vi "convertPhysicalChannels.vi"(8 "error in (no error)":errorcluster, 10 "physicalChannels":string[](array[string]), 11 "K2602 in":refnum<class "K2602.lvclass">) -> (0 "error out":errorcluster, 2 "channel":i32[](array[numeric]), 3 "K2602 out":refnum<class "K2602.lvclass">)   [LabVIEW 2011, in "Hardware.lvlib" / "Channels.lvlib" / "K2602.lvclass"]
uses:
  K2602.lvclass
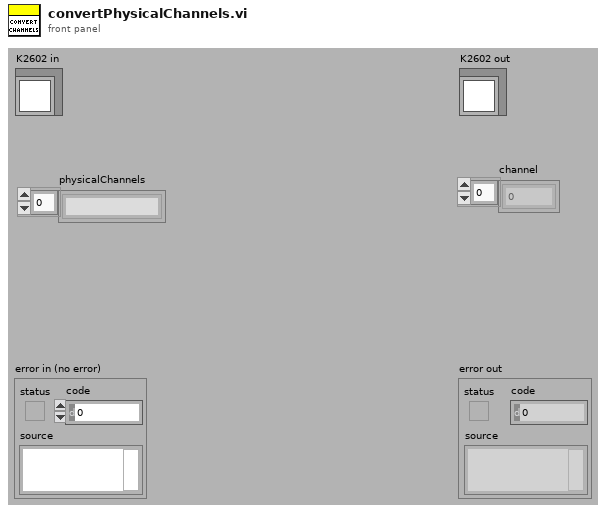
[diagram p1: front panel]
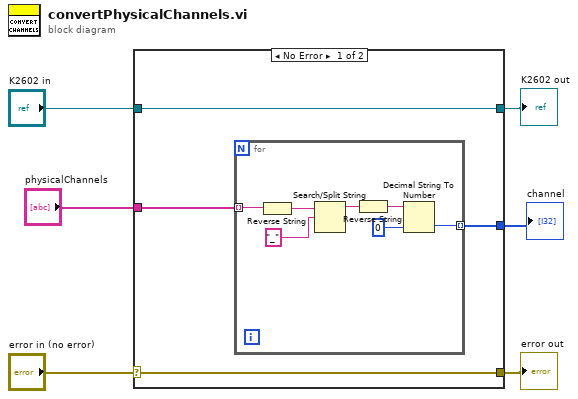
[diagram p0: block diagram]
diagram:
  n1 = case shown="No Error" "error in (no error)" {
    selector: "error in (no error)" -> [w9 w19]
    tunnel: [w9 w19] -> w5
    tunnel: [w10 w18] -> w3
    tunnel: "K2602 in" -> [w10 w18]
    tunnel: "physicalChannels" -> [w8 _]
    tunnel: [w7 _] -> w1
    frame No Error {
      n2 = for {
        tunnel: w8 -> [w17] mode=indexing
        tunnel: [w12] -> w7 mode=indexing
        n3 = Reverse String(1:w17) -> (0:w16:string)
        n4 = Search/Split String(string=w16, search string/char (-)="_") -> (substring before match=w14:string)  [unwired: 1 in, 2 out]
        n5 = Reverse String(1:w14) -> (0:w13:string)
        n6 = Decimal String To Number(string=w13, default (0L)=0) -> (number=w12:i32)  [unwired: 1 in, 1 out]
      }
    }
    frame Error {
    }
  }
  "error out" <- w5
  "K2602 out" <- w3
  "channel" <- w1
